vi "SEMA2.vi"() -> ()   [LabVIEW 2013]
panel:
  out "B":bool=TRUE
  out "A":bool
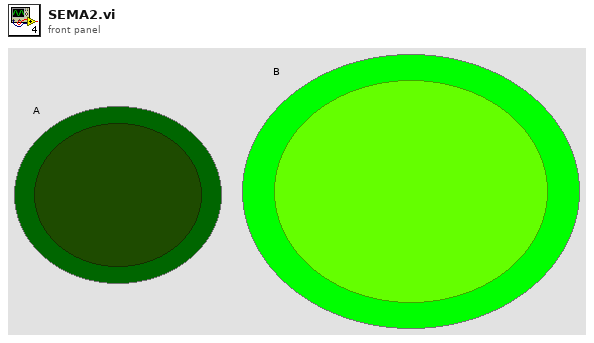
[diagram p1: front panel]
types:
  T1 = typedef "Semaphore RefNum" = refnum<k1>
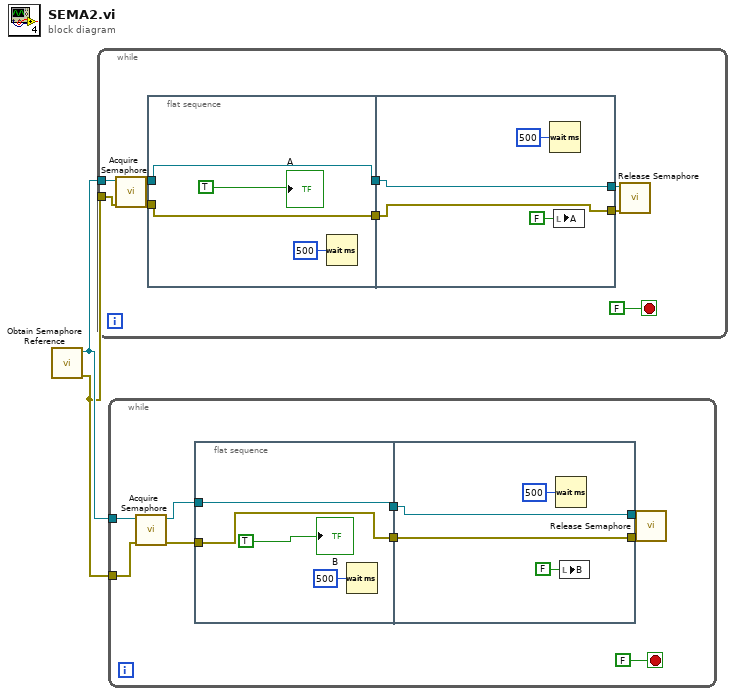
[diagram p0: block diagram]
diagram:
  n1 = call <vilib>:"Obtain Semaphore Reference.vi"() -> ("error out"=w1:errorcluster, "semaphore"=w2:T1)  [unwired: 5 in, 1 out]
  n2 = while {
    tunnel: w2 -> [w10]
    tunnel: w1 -> [w3]
    stop <- FALSE stop-if-true
    n3 = call <vilib>:"Acquire Semaphore.vi"("error in (no error)"=w3, "semaphore"=w10) -> ("error out"=w5:errorcluster, "semaphore out"=w8:T1)  [unwired: 3 in, 1 out]
    n4 = flat-sequence {
      tunnel: [w13] -> w9
      tunnel: w8 -> [w13]
      tunnel: [w12] -> w6
      tunnel: w5 -> [w12]
      tunnel: w9 -> [w17]
      tunnel: [w17] -> w7
      tunnel: w6 -> [w16]
      tunnel: [w16] -> w4
      frame #0 {
        n5 = Wait (ms)(milliseconds to wait=u32 500) -> ()  [unwired: 1 out]
        "A" <- TRUE
      }
      frame #1 {
        n6 = Wait (ms)(milliseconds to wait=u32 500) -> ()  [unwired: 1 out]
        n7 = local write "A"(FALSE ("A")) -> ()
      }
    }
    n8 = call <vilib>:"Release Semaphore.vi"("error in (no error)"=w4, "semaphore"=w7) -> ()  [unwired: 4 in, 2 out]
  }
  n9 = while {
    tunnel: w2 -> [w27]
    tunnel: w1 -> [w26]
    stop <- FALSE stop-if-true
    n10 = call <vilib>:"Acquire Semaphore.vi"("error in (no error)"=w26, "semaphore"=w27) -> ("error out"=w22:errorcluster, "semaphore out"=w24:T1)  [unwired: 3 in, 1 out]
    n11 = flat-sequence {
      tunnel: [w30] -> w25
      tunnel: w24 -> [w30]
      tunnel: [w29] -> w23
      tunnel: w22 -> [w29]
      tunnel: w25 -> [w34]
      tunnel: w23 -> [w33]
      tunnel: [w34] -> w21
      tunnel: [w33] -> w20
      frame #0 {
        n12 = Wait (ms)(milliseconds to wait=u32 500) -> ()  [unwired: 1 out]
        "B" <- TRUE
      }
      frame #1 {
        n13 = Wait (ms)(milliseconds to wait=u32 500) -> ()  [unwired: 1 out]
        n14 = local write "B"(FALSE ("B")) -> ()
      }
    }
    n15 = call <vilib>:"Release Semaphore.vi"("error in (no error)"=w20, "semaphore"=w21) -> ()  [unwired: 4 in, 2 out]
  }
